vi "WorkorderHandler_getObjectReference.vi"(0 "object name":string, 5 "error in (no error)":errorcluster) -> (14 "reference":T1, 19 "error out":errorcluster)   [LabVIEW 2011]
doc: "Looks up an existing dqGOOP object with object name and returns a refnum"
uses:
  DataStructures/WorkorderHandler_ObjectReference.ctl
panel:
  in  "reference (default)":T1
  # "Copyright (C) 2004 DataAct Incorporated"
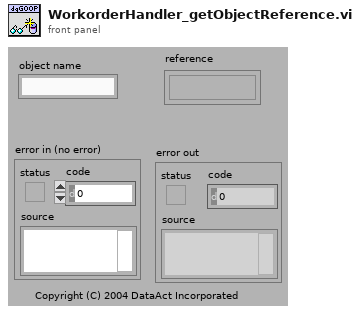
[diagram p1: front panel]
types:
  T1 = typedef "WorkorderHandler_ObjectReference.ctl" = refnum<k1>
  T2 = typedef "WorkorderHandler_ObjectData.ctl" = cluster{"Table":string[][], "Script":string, "Order":string, "No":string, "Time":dbl}
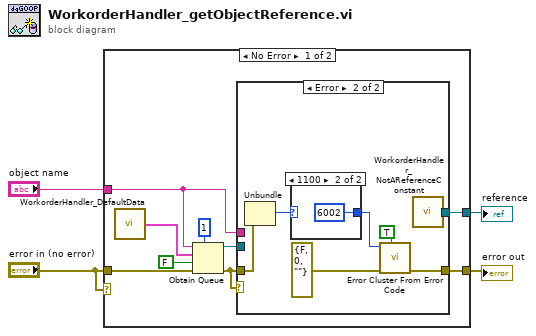
[diagram p0: block diagram]
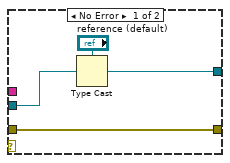
[diagram p2: hidden frame]
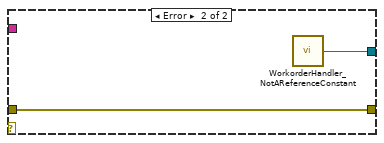
[diagram p4: hidden frame]
diagram:
  n1 = case shown="No Error" "error in (no error)" {
    tunnel: [w11 w27] -> w4
    tunnel: [w8 w28] -> w3
    tunnel: "error in (no error)" -> [w7 w27]
    tunnel: "object name" -> [w5 _]
    frame No Error {
      n2 = call "WorkorderHandler_DefaultData.vi"() -> ("data"=w9:T2)
      n3 = Obtain Queue(max queue size (-1, unlimited)=1, name (unnamed)=w5, element data type=w9, create if not found? (T)=FALSE, error in (no error)=w7) -> (queue out=w13:refnum<queue>, error out=w6:errorcluster)  [unwired: 1 out]
      n4 = case shown="Error" w6 {
        tunnel: w13 -> [w15 _]
        tunnel: [w17 w18] -> w11
        tunnel: w5 -> [_ _]
        tunnel: [w14 w24] -> w8
        tunnel: w6 -> [w17 w23]
        frame No Error {
          n5 = Type Cast(type="reference (default)", x=w15) -> (*(type *) &x=w14:T1)
        }
        frame Error {
          n6 = Unbundle(w23) -> ("code"=w22:i32)  [unwired: 2 out]
          n7 = case shown="1100" w22 {
            selector: w22 -> [w25 _]
            tunnel: [w25 6002 ("code")] -> w20
            frame Default {
            }
            frame 1100 {
            }
          }
          n8 = call <vilib>:"Error Cluster From Error Code.vi"("show call chain? (False)"=TRUE, "error in (no error)"=errorcluster {"status"=FALSE, "code"=0, "source"=""} ("error out"), "error code (0)"=w20) -> ("error out"=w18:errorcluster)  [unwired: 6 out]
          n9 = call "WorkorderHandler_NotAReferenceConstant.vi"() -> ("reference"=w24:T1)
        }
      }
    }
    frame Error {
      n10 = call "WorkorderHandler_NotAReferenceConstant.vi"() -> ("reference"=w28:T1)
    }
  }
  "error out" <- w4
  "reference" <- w3
